vi "File_Save png Glyph.vi"(8 "Error":errorcluster, 10 "Glyph Data":T1, 11 "Starting Folder":path) -> (0 "Error Out":errorcluster)   [LabVIEW 2021]
uses:
  TypeDefs/Cluster_Glyph Data.ctl
  vi.lib/LabVIEW Icon API/lv_icon/lv_icon.lvlib
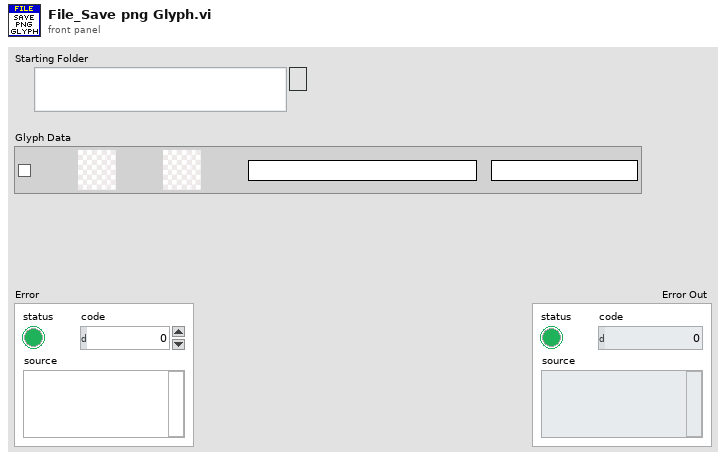
[diagram p1: front panel]
types:
  T1 = typedef "Cluster_Glyph Data.ctl" = cluster{"Install":bool, "Current":picture, "Icon Library":picture, "Subfolder":string, "Name":string}
  T2 = typedef "imagedata.ctl" = cluster{"image type":i32, "image depth":i32, "image":u8[], "mask":u8[], "colors":u32[], "Rectangle":cluster{"left":i16, "top":i16, "right":i16, "bottom":i16}}
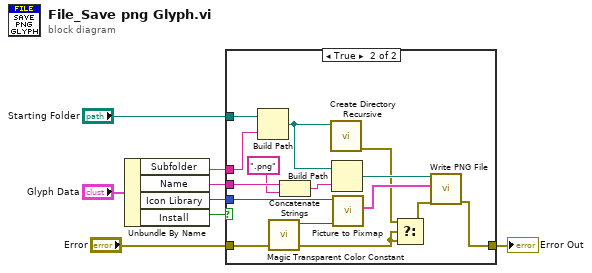
[diagram p0: block diagram]
diagram:
  n1 = Unbundle By Name("Glyph Data") -> ("Subfolder"=w5:string, "Name"=w4:string, "Icon Library"=w3:picture, "Install"=w2:bool)
  n2 = case shown="True" w2 {
    tunnel: w3 -> [_ w20]
    tunnel: w4 -> [_ w18]
    tunnel: w5 -> [_ w22]
    tunnel: "Starting Folder" -> [_ w23]
    tunnel: "Error" -> [w9 w14]
    tunnel: [w9 w15] -> w8
    frame False {
    }
    frame True {
      n3 = Build Path(base path=w23, name or relative path=w22) -> (appended path=w11:path)
      n4 = call "Magic Transparent Color Constant.vi"() -> ("Magic transparent color constant"=w12:u32)  [unwired: 11 out]
      n5 = Concatenate Strings(w18, ".png" ("string")) -> (w16:string)
      n6 = call <vilib>:"Create Directory Recursive.vi"("directory"=w11) -> ("error out"=w10:errorcluster)  [unwired: 2 in, 4 out]
      n7 = Build Path(base path=w11, name or relative path=w16) -> (appended path=w19:path)
      n8 = call <vilib>:"Picture to Pixmap.vi"("Background Color"=w12, "picture"=w20) -> ("image data"=w21:T2)  [unwired: 2 in, 7 out]
      n9 = Select(t=w10, s=w14, f=w14) -> (s? t:f=w13:errorcluster)
      n10 = call <vilib>:"Write PNG File.vi"("error in (no error)"=w13, "image data"=w21, "path to PNG file"=w19) -> ("error out"=w15:errorcluster)  [unwired: 8 out]
    }
  }
  "Error Out" <- w8
